vi "求最大值最小值-for.vi"() -> ()   [LabVIEW 2012]
panel:
  out "波形图表":dbl(graph)
  out "最小值":dbl
  out "最大值":dbl
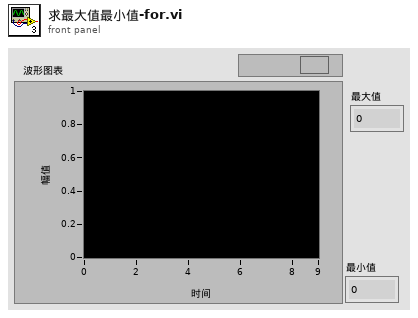
[diagram p1: front panel]
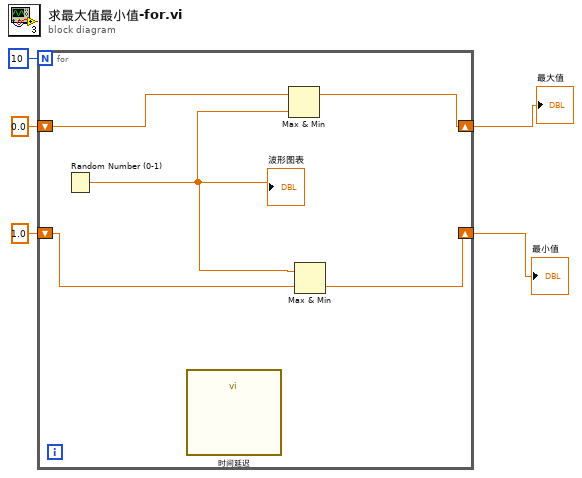
[diagram p0: block diagram]
diagram:
  n1 = for {
    N: 10 -> [_]
    shift-right: [w7] -> w4
    shift-left: 0.0 -> [w10]
    shift-right: [w6] -> w3
    shift-left: 1.0 -> [w8]
    n2 = Random Number (0-1)() -> (number: 0 to 1=w9:dbl)
    "波形图表" <- w9
    n3 = call "时间延迟"() -> ()  [unwired: 11 in, 1 out]
    n4 = Max & Min(x=w10, y=w9) -> (max(x,y)=w7:dbl)  [unwired: 1 out]
    n5 = Max & Min(x=w9, y=w8) -> (min(x,y)=w6:dbl)  [unwired: 1 out]
  }
  "最大值" <- w4
  "最小值" <- w3
